vi "ini_sesion.vi"(8 "error in (no error)":errorcluster, 11 "USRP_1_x_200MHz in":refnum<class "USRP_1_x_200MHz.lvclass">) -> (0 "error out":errorcluster, 3 "USRP_1_x_200MHz out":refnum<class "USRP_1_x_200MHz.lvclass">)   [LabVIEW 2021, in "USRP_1_x_200MHz.lvclass"]
uses:
  USRP_1_x_200MHz.lvclass
  USRP_1_x_200MHz.lvclass/USRP_1_x_200MHz.ctl
  <vilib>/rvi/interface/nirviOpenFPGA/nirviOpenFPGA.xnode
  FPGA Bitfiles/pulse_Tx_one_channel.lvbitx
  <vilib>/rvi/interface/nirviMethod/nirviMethod.xnode
  <vilib>/FPGAPlugInAG/Dynamic/niLvFpga_ConfigureFifo_Dynamic.vi
  <vilib>/rvi/errors/niLvFpgaMergeErrorWithErrorCode.vi
  <vilib>/rvi/interface/nirviReadWriteControl/nirviReadWriteControl.xnode
  NiFpgaLv.dll
  <vilib>/Utility/error.llb/Error Cluster From Error Code.vi
  <vilib>/rvi/interface/Simulation/niFpgaSimulationCallBeginRW.vi
  <vilib>/rvi/errors/niLvFpgaAdjustHostInterfaceError.vi
  <instrlib>/niUsrpRio/Config/v1/Host/Private/LO Source.ctl
  <instrlib>/niUsrpRio/Config/v1/Host/niUsrpRio Config v1 Host.lvlib
  <vilib>/FPGAPlugInAG/USRP 294xR; 295xR 200 MSps/niLvFpga_Open_USRP 294xR; 295xR 200 MSps.vi
  <vilib>/rvi/interface/common/dynamic/niFpgaDynamicAddResources.vi
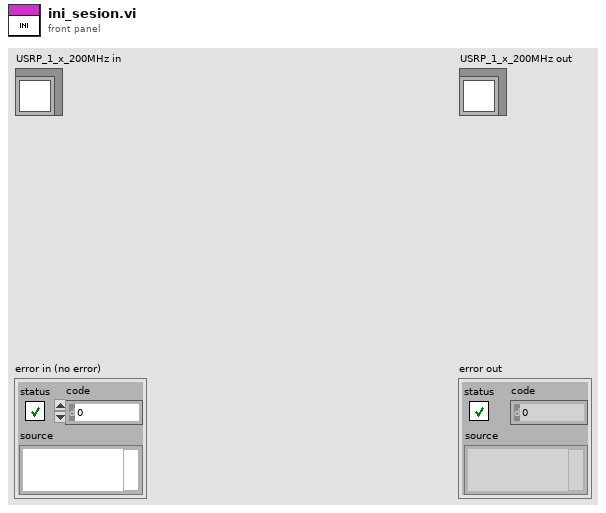
[diagram p1: front panel]
types:
  T1 = cluster{"gain I":fxp<+/-,24,3>, "gain Q":fxp<+/-,24,3>}
  T2 = typedef "niUsrpRio Config v1 Host.lvlib/LO Source.ctl" = enum16{"Internal", "Companion", "External", "Reimport"}
  T3 = typedef "nirio_resource_hc.ctl" = tag
  T4 = typedef "niUsrpRio Config v1 Host.lvlib/niUsrpRio Session.ctl" = cluster{"FPGA Interface":refnum<k20>, "RIO Interface Number":u32, "Data Clock Rate":u32, "FPGA Data Clock Rate":u32, "Global Settings Register Bus":T5, "Radio 0 Settings Register Bus":T5, "Radio 1 Settings Register Bus":T5, "Radio Settings Bus Semaphore":T6, "DB Queues":T7[], "Characterization Data Valid?":bool, "EEPROM Header":T8, "Device Data Header":T9, "EEPROM Characterization Header":T10, "Characterization Data":T11[], "FPGA Current Version":u32, "FPGA Oldest Compatible Version":u32, "Fixed Logic Current Version":u32, "Fixed Logic Oldest Compatible Version":u32, "FPGA Radio Settings Bus Current Version":u32, "FPGA Radio Settings Bus Oldest Compatible Version":u32, "FPGA Board Config Current Version":u32, "FPGA Board Config Oldest Compatible Version":u32, "Daughterboard Clock Rate":u32, "daughterboard configuration session handles":u64[]}
  T5 = typedef "niInstr Register Bus v0 Host.lvlib/Register Bus Session.ctl" = refnum<queue>
  T6 = typedef "Semaphore RefNum" = refnum<k1>
  T7 = typedef "niUsrpRio Config v1 Host.lvlib/DB Queue Reference.ctl" = refnum<queue>
  T8 = typedef "niUsrpRio Config v1 Host.lvlib/EEPROM Header.ctl" = cluster{"Checksum":u32, "Product Code":u16, "Hardware Current Version":u16, "Hardware Oldest Compatible Version":u16, "EEPROM Map Current Version":u16, "EEPROM Map Oldest Compatible Version":u16, "User Password":string, "Pointer to Factory Header":u32, "Pointer to User Header":u32, "Recommended Interval":u16, "Number of Reserved Bytes":i32, "Number of Daughterboards":u8, "Daughterboard IDs":u16[], "Daughterboard Serial Numbers":string[]}
  T9 = typedef "niUsrpRio Config v1 Host.lvlib/EEPROM Device Data Header.ctl" = cluster{"Checksum":u32, "Number of Channels":u8, "Number of Gain Settings":u16[], "Pointer to Characterization Data":u32[], "Number of Reserved Bytes":i32, "Number of Frequencies":u16[]}
  T10 = typedef "niUsrpRio Config v1 Host.lvlib/EEPROM Characterization Header.ctl" = cluster{"Checksum":u32, "Date":timestamp, "Temperature":sgl, "Misc. Info":string, "Pointer to Device Data Header":u32, "Number of Reserved Bytes":i32}
  T11 = typedef "niUsrpRio Config v1 Host.lvlib/Characterization Data.ctl" = cluster{"Gains[dB]":dbl[], "Frequencies [Hz]":dbl[], "IQ Imbalance Table":T12[], "Measured Gains[dB]":dbl[][]}
  T12 = typedef "niUsrpRio Config v1 Host.lvlib/IQ Imbalance.ctl" = cluster{"Gain Imbalance [linear]":dbl, "Phase Imbalance [radians]":dbl, "Offset":cdb}
  T13 = typedef "niInstr DSP v1 Shared.lvlib/IQ Impairments.ctl" = cluster{"inline gain I":fxp<+/-,18,1>, "inline gain Q":fxp<+/-,18,1>, "cross gain I":fxp<+/-,18,1>, "cross gain Q":fxp<+/-,18,1>, "pre-gain offset I":fxp<+/-,18,1>, "pre-gain offset Q":fxp<+/-,18,1>, "post-gain offset I":fxp<+/-,18,1>, "post-gain offset Q":fxp<+/-,18,1>}
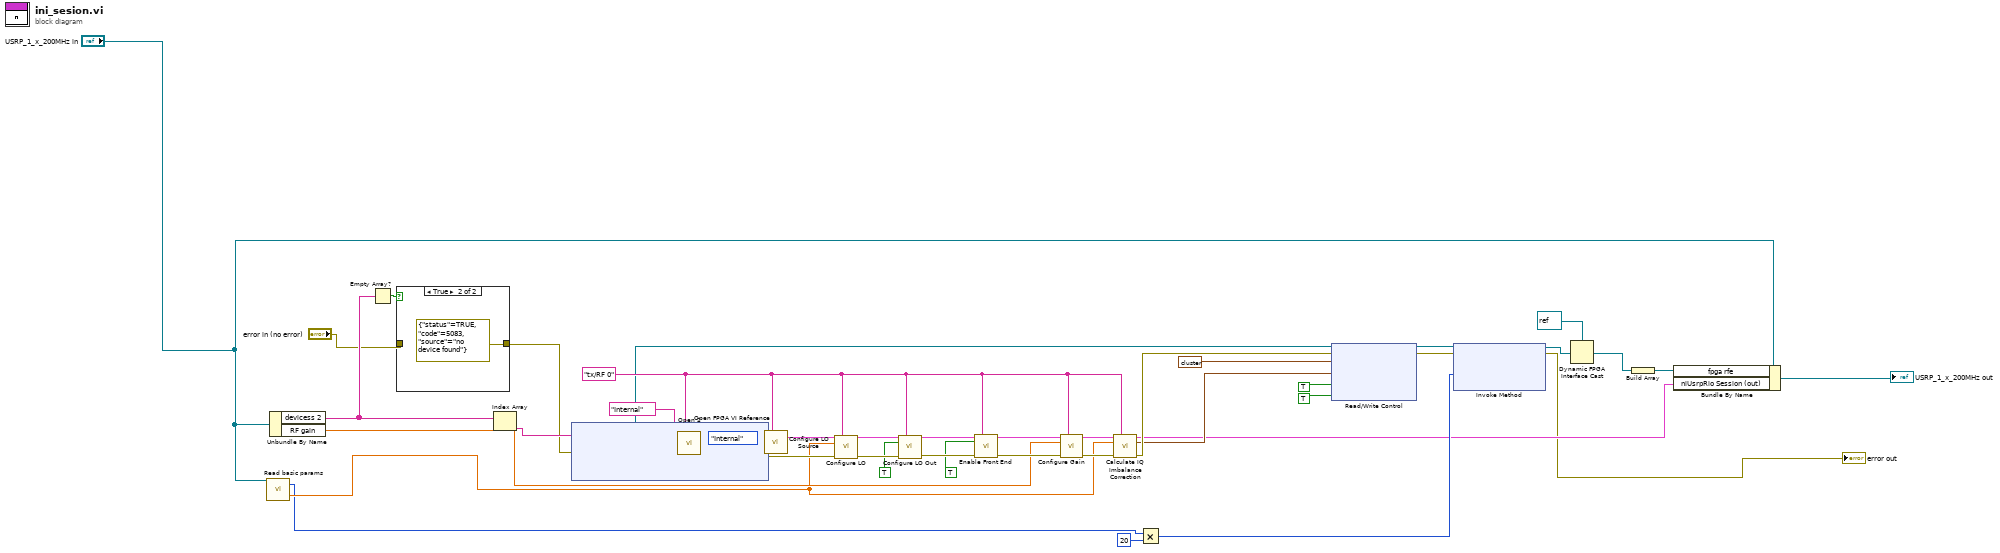
[diagram p0: block diagram]
diagram:
  w19 = "tx/RF 0" ("scope")
  n1 = call-dynamic "Read basic params.vi"("device_type in"="USRP_1_x_200MHz in") -> ("buffer size"=w3:u32, "center frequency (Hz)"=w4:dbl)  [unwired: 13 in, 4 out]
  n2 = Unbundle By Name("USRP_1_x_200MHz in") -> ("devicess 2"=w8:T3[], "RF gain"=w10:dbl)
  n3 = Empty Array?(array=w8) -> (empty?=w9:bool)
  n4 = case shown="True" w9 {
    tunnel: [w45 errorcluster {"status"=TRUE, "code"=5083, "source"="no device found"} ("error in (no error)")] -> w7
    tunnel: "error in (no error)" -> [w45 _]
    frame False {
    }
    frame True {
    }
  }
  n5 = Index Array(array=w8) -> (element=w39:T3)  [unwired: 1 in]
  n6 = xnode ("Open FPGA VI Reference")("error in"=w7, "resource name"=w39) -> ("FPGA VI Reference Out"=w18:refnum<k20>, "error out"=w40:errorcluster)
  n7 = call <instrlib>:"Open 2.vi"("fpga ref"=w18, "scope"=w19, "Reference Frequency Source"="Internal", "error in"=w40) -> ("niUsrpRio Session (out)"=w41:T4, "error out"=w43:errorcluster)  [unwired: 10 in]
  n8 = call <instrlib>:"Configure LO Source.vi"("niUsrpRio Session"=w41, "scope"=w19, "lo source"=LO_Source."Internal", "error in"=w43) -> ("niUsrpRio Session (out)"=w21:T4, "error out"=w20:errorcluster)  [unwired: 10 in]
  n9 = call <instrlib>:"Configure LO.vi"("niUsrpRio Session"=w21, "scope"=w19, "frequency"=w4, "error in"=w20) -> ("niUsrpRio Session (out)"=w38:T4, "error out"=w37:errorcluster)  [unwired: 8 in, 2 out]
  n10 = call <instrlib>:"Configure LO Out.vi"("niUsrpRio Session"=w38, "scope"=w19, "enable"=TRUE ("enable 0"), "error in"=w37) -> ("niUsrpRio Session (out)"=w35:T4, "error out"=w32:errorcluster)  [unwired: 10 in]
  n11 = call <instrlib>:"Enable Front End.vi"("niUsrpRio Session"=w35, "scope"=w19, "enable"=TRUE ("enable 0 2"), "error in"=w32) -> ("niUsrpRio Session (out)"=w34:T4, "error out"=w33:errorcluster)  [unwired: 10 in]
  n12 = call <instrlib>:"Configure Gain.vi"("niUsrpRio Session"=w34, "scope"=w19, "gain"=w10, "error in"=w33) -> ("niUsrpRio Session (out)"=w30:T4, "error out"=w29:errorcluster)  [unwired: 9 in, 1 out]
  n13 = call <instrlib>:"Calculate IQ Imbalance Correction.vi"("niUsrpRio Session"=w30, "scope"=w19, "frequency"=w4, "error in"=w29) -> ("niUsrpRio Session (out)"=w11:T4, "IQ imbalance correction"=w25:T13, "error out"=w28:errorcluster)  [unwired: 8 in, 1 out]
  n14 = Multiply(x=w3, y=u32 20) -> (x*y=w15:u32)
  n15 = xnode ("Read/Write Control")("FPGA VI Reference In"=w18, "error in"=w28, "tx.gain.0"=T1 {"gain I"=1.0, "gain Q"=1.0}, "tx.impairments.0"=w25, "reset system clock"=TRUE, "RF 0/Tx/Enable"=TRUE) -> ("FPGA VI Reference Out"=w23:refnum<k20>, "error out"=w22:errorcluster)
  n16 = xnode ("Invoke Method")("FPGA VI Reference In"=w23, "error in"=w22, "Requested Depth"=w15) -> ("FPGA VI Reference Out"=w17:refnum<k20>, "error out"=→"error out":errorcluster)  [unwired: 1 out]
  n17 = Dynamic FPGA Interface Cast(Session In=refnum<k20> refnum ("fpga interface out"), Type=w17) -> (Session Out=w13:refnum<k20>)
  n18 = Build Array(w13) -> (w12:refnum<k20>[])
  n19 = Bundle By Name(cluster="USRP_1_x_200MHz in", "fpga rfe"=w12, "niUsrpRio Session (out)"=w11) -> (→"USRP_1_x_200MHz out":refnum<class "USRP_1_x_200MHz.lvclass">)
